vi "Trap Pos RMS.vi"(3 "Accumulated array":dbl[][](array[numeric]), 4 "New Array":dbl[][](array[numeric]), 5 "Number of sets to average":dbl) -> (0 "Output accumulated array":dbl[][](array[numeric]), 1 "RMS":dbl[](array[numeric]), 2 "Mean":dbl[](array[numeric]))   [LabVIEW 2014]
uses:
  <vilib>/Analysis/baseanly.llb/Mean (DBL).vi
  <vilib>/Analysis/NI_AALBase.lvlib
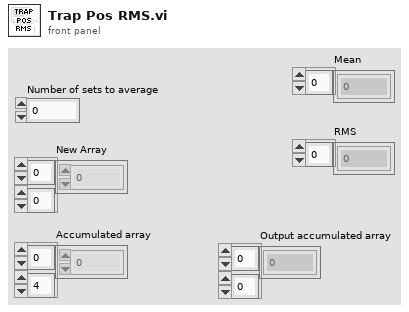
[diagram p1: front panel]
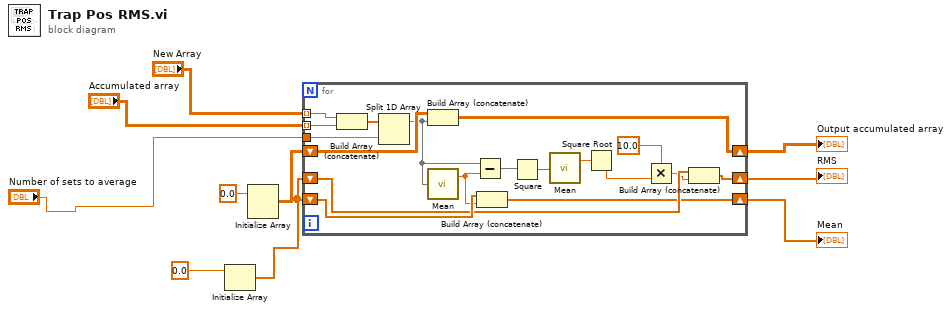
[diagram p0: block diagram]
diagram:
  n1 = Initialize Array(0.0) -> (w5:dbl[])  [unwired: 1 in]
  n2 = Initialize Array(0.0) -> (w9:dbl[][])  [unwired: 2 in]
  n3 = for {
    tunnel: "New Array" -> [w28] mode=indexing
    tunnel: "Accumulated array" -> [w27] mode=indexing
    tunnel: "Number of sets to average" -> [w26]
    shift-right: [w19] -> w6
    shift-left: w9 -> [w18]
    shift-right: [w14] -> w8
    shift-left: w5 -> [w17]
    shift-right: [w13] -> w7
    shift-left: w5 -> [w16]
    n4 = Build Array (concatenate)(w28, w27) -> (w25:dbl[])
    n5 = Split 1D Array(array=w25, index=w26) -> (first subarray=w12:dbl[])  [unwired: 1 out]
    n6 = Build Array (concatenate)(w18, w12) -> (w19:dbl[][])
    n7 = call-poly <vilib>:"Mean.vi"("X"=w12) -> ("mean"=w11:dbl)  [unwired: 1 out]
    n8 = Subtract(x=w12, y=w11) -> (x-y=w20:dbl[])
    n9 = Build Array (concatenate)(w17, w11) -> (w14:dbl[])
    n10 = Square(x=w20) -> (x^2=w21:dbl[])
    n11 = call-poly <vilib>:"Mean.vi"("X"=w21) -> ("mean"=w22:dbl)  [unwired: 1 out]
    n12 = Square Root(x=w22) -> (sqrt(x)=w23:dbl)
    n13 = Multiply(x=10.0, y=w23) -> (x*y=w15:dbl)
    n14 = Build Array (concatenate)(w16, w15) -> (w13:dbl[])
  }
  "Output accumulated array" <- w6
  "Mean" <- w8
  "RMS" <- w7
